vi "Create Channel Name.vi"(8 "error in":errorcluster, 9 "Channel Name":string, 10 "Plugin Name":string) -> (0 "error out":errorcluster, 1 "Data Channel Name":string)   [LabVIEW 2023, in "Utilities.lvlib"]
uses:
  Utilities.lvlib
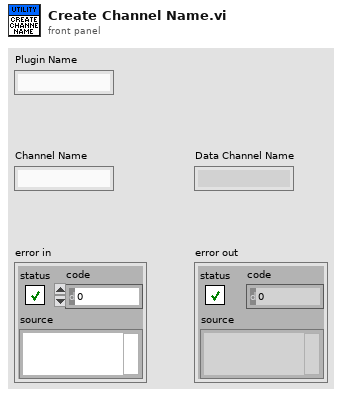
[diagram p1: front panel]
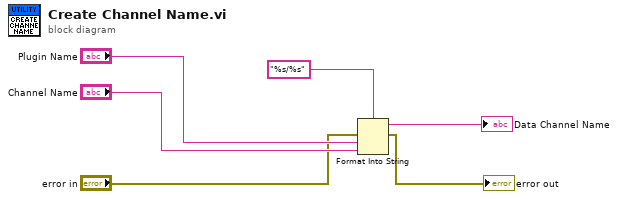
[diagram p0: block diagram]
diagram:
  n1 = Format Into String(format string="%s/%s", error in="error in", "Plugin Name", "Channel Name") -> (resulting string=→"Data Channel Name":string, error out=→"error out":errorcluster)  [unwired: 1 in]
